vi "Clear.vi"(8 "error in (no error)":errorcluster, 10 "Session In":refnum<class "Session.lvclass">, 11 "Character LCD in":refnum<class "Grove I2C LCD.lvclass">) -> (0 "error out":errorcluster, 2 "Session Out":refnum<class "Session.lvclass">, 3 "Character LCD out":refnum<class "Grove I2C LCD.lvclass">)   [LabVIEW 2020, in "CTI-Peripheral.lvlib" / "Grove I2C LCD.lvclass"]
uses:
  Grove I2C LCD.lvclass
  CTI/Session/Session.lvclass
  HD44780 LCD/Command.ctl
  2887e299-174e-4799-904e-3631b3a1dc1e.vi
  HD44780 LCD/HD44780 LCD.lvlib
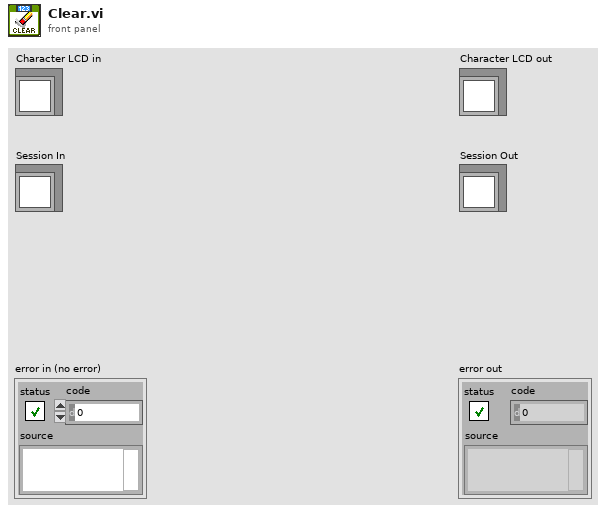
[diagram p1: front panel]
types:
  T1 = typedef "CTI-Peripheral.lvlib/HD44780 LCD.lvlib/Command.ctl" = enum16{"ClearDisplay", "ReturnHome", "EntryModeSet", "DisplayControl", "CursorShift", "FunctionSet", "SetCGRamAddr", "SetDDRamAddr"}
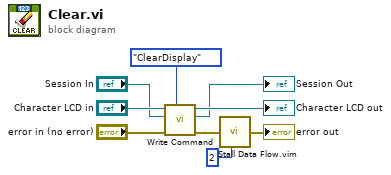
[diagram p0: block diagram]
diagram:
  n1 = call "Write Command.vi"("Command"=Command."ClearDisplay", "error in (no error)"="error in (no error)", "Session In"="Session In", "Grove I2C LCD in"="Character LCD in") -> ("error out"=w8:errorcluster, "Session Out"=→"Session Out":refnum<class "Session.lvclass">, "Grove I2C LCD out"=→"Character LCD out":refnum<class "Grove I2C LCD.lvclass">)  [unwired: 5 in]
  n2 = call "Stall Data Flow.vim"("value in"=w8, "milliseconds to wait"=u32 2) -> ("value out"=→"error out":errorcluster)  [unwired: 1 out]
